vi "ParseOutput.vi"(8 "error in (no error)":errorcluster, 10 "JUnit report path":path, 11 "utf results in":T1[](array[typedef])) -> (0 "error out":errorcluster, 2 "Passed?":bool, 3 "Output":string)   [LabVIEW 2014, in "RunUnitTests.lvclass"]
uses:
  RunUnitTests.lvclass
  <vilib>/utf/common/utf_test_result_testfile.ctl
  <vilib>/utf/common/utf_test_result_testcase.ctl
  <vilib>/utf/common/utf_test_result.ctl
  <vilib>/utf/common/utf_test_result_troll_new.ctl
  <vilib>/utf/common/utf_vector_result.ctl
  <vilib>/utf/common/utf_test_result_failure.ctl
  <vilib>/utf/common/utf_test_comparison_operators.ctl
  <vilib>/utf/common/utf_vi_tag.ctl
  <vilib>/utf/common/utf_test_result_input_data.ctl
  <vilib>/utf/common/utf_code_coverage.ctl
  <vilib>/utf/common/utf_error_data.ctl
  <vilib>/utf/common/utf_error_type.ctl
  <vilib>/utf/common/utf_subvi_info.ctl
  <vilib>/utf/NI_UnitTestFramework.lvlib
panel:
  in  "JUnit report path infromation":string="Please find the JUnit report path at \"%s\"."
  in  "No of test path not processed":string="%d tests path not processed.\\n"
  in  "No of test path skipped":string="%d tests path skipped.\\n"
  in  "No of test path errored":string="%d tests path errored.\\n"
  in  "No of test path failed":string="%d tests path failed.\\n"
  in  "Number of test path passed":string="%d tests path passed.\\n"
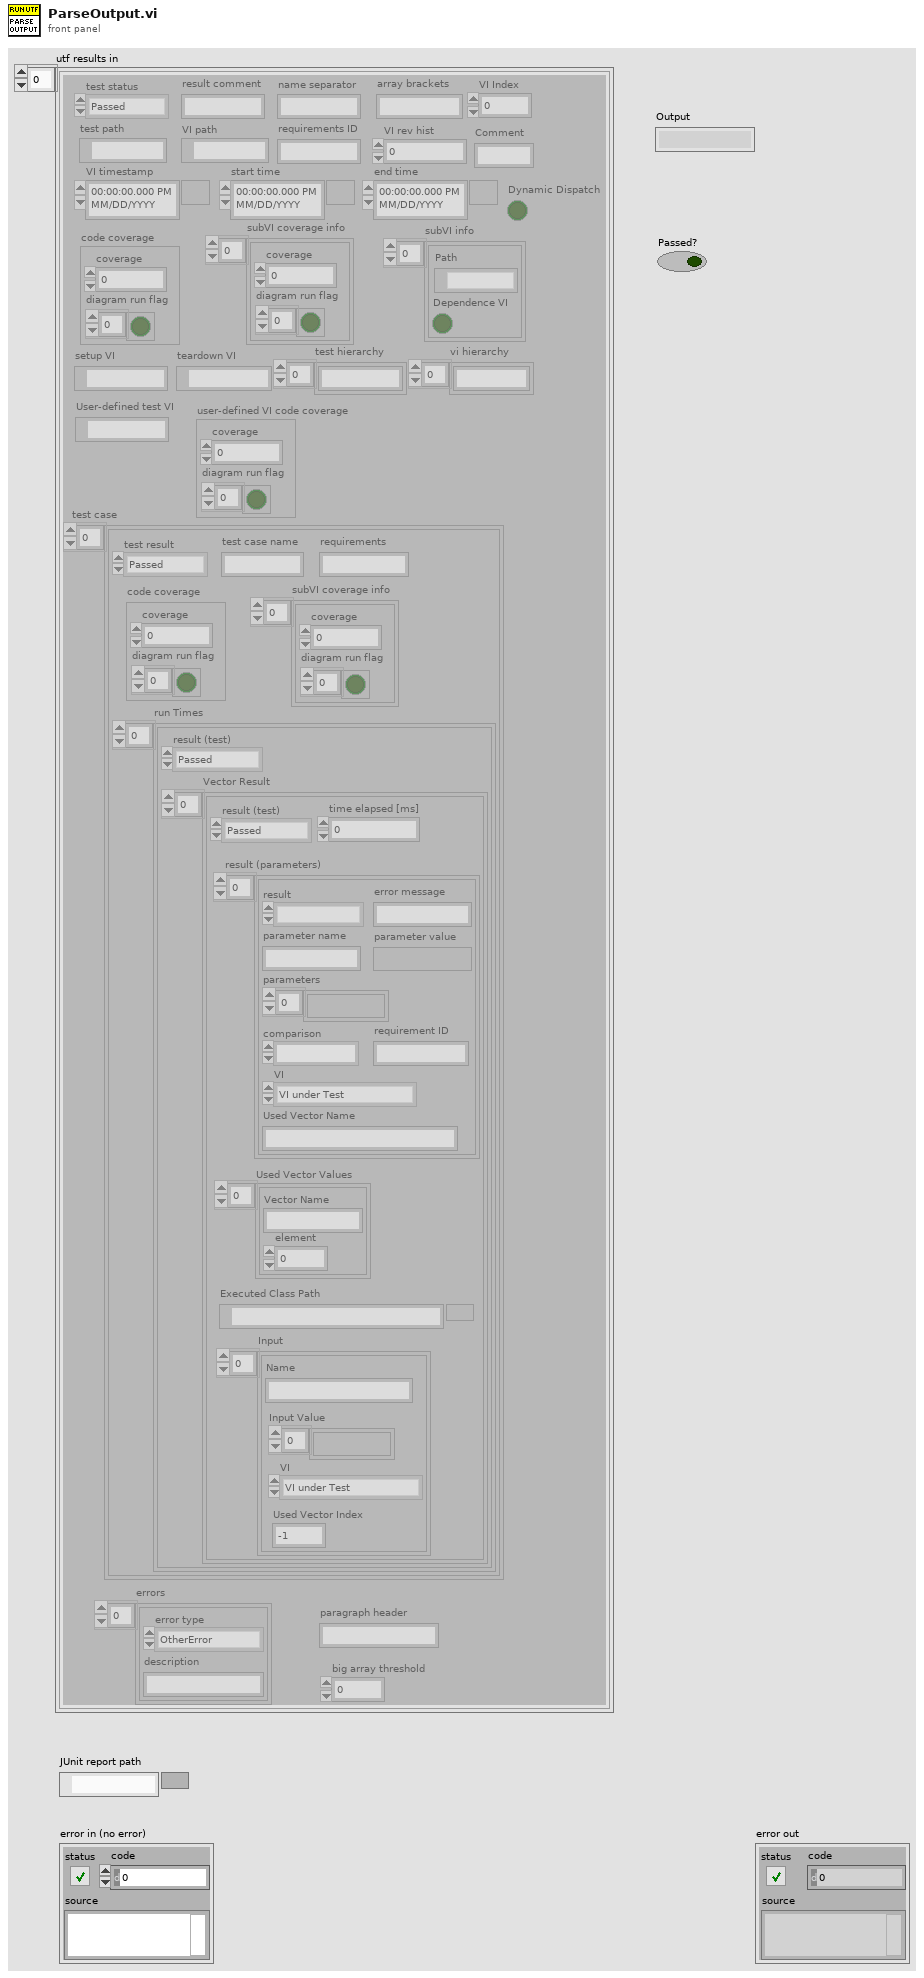
[diagram p1: front panel]
types:
  T1 = typedef "NI_UnitTestFramework.lvlib/utf_test_result_testfile.ctl" = cluster{"test case":T2[], "test status":T3, "test path":path, "setup VI":path, "teardown VI":path, "code coverage":T10, "start time":timestamp, "end time":timestamp, "test hierarchy":string[], "VI path":path, "VI timestamp":timestamp, "VI rev hist":i32, "requirements ID":string, "array brackets":string, "name separator":string, "errors":T11[], "paragraph header":string, "result comment":string, "vi hierarchy":string[], "subVI coverage info":T10[], "subVI info":T13[], "big array threshold":u32, "VI Index":i32, "Comment":string, "Dynamic Dispatch":bool, "User-defined test VI":path, "user-defined VI code coverage":T10}
  T2 = typedef "NI_UnitTestFramework.lvlib/utf_test_result_testcase.ctl" = cluster{"test result":T3, "run Times":T4[], "test case name":string, "requirements":string, "code coverage":T10, "subVI coverage info":T10[]}
  T3 = typedef "NI_UnitTestFramework.lvlib/utf_test_result.ctl" = enum16{"Passed", "Failed", "Error", "Skipped", "Not Processed"}
  T4 = typedef "NI_UnitTestFramework.lvlib/utf_test_result_troll_new.ctl" = cluster{"result (test)":T3, "Vector Result":T5[]}
  T5 = typedef "NI_UnitTestFramework.lvlib/utf_vector_result.ctl" = cluster{"time elapsed [ms]":u32, "result (test)":T3, "result (parameters)":T6[], "Used Vector Values":cluster{"Vector Name":string, "element":i32}[], "Executed Class Path":path, "Input":T9[]}
  T6 = typedef "NI_UnitTestFramework.lvlib/utf_test_result_failure.ctl" = cluster{"result":T3, "error message":string, "parameter name":string, "parameter value":variant, "parameters":variant[], "comparison":T7, "requirement ID":string, "VI":T8, "Used Vector Name":string}
  T7 = typedef "NI_UnitTestFramework.lvlib/utf_test_comparison_operators.ctl" = enum16{"=", "!=", ">", ">=", "<", "<=", "range", "symmetric tolerance", "asymmetric tolerance", "string contains", "string not contain", "array size", "string length", "array range", "by element", "array range (limit array)", "user-defined", "array contains", "array not contain", "vector length", "= (elm)", "!= (elm)", "= (case insensitive)", "!= (case insensitive)"}
  T8 = typedef "NI_UnitTestFramework.lvlib/utf_vi_tag.ctl" = enum16{"Setup VI", "VI under Test", "Teardown VI"}
  T9 = typedef "NI_UnitTestFramework.lvlib/utf_test_result_input_data.ctl" = cluster{"Name":string, "Input Value":variant[], "VI":T8, "Used Vector Index":i32}
  T10 = typedef "NI_UnitTestFramework.lvlib/utf_code_coverage.ctl" = cluster{"coverage":dbl, "diagram run flag":bool[]}
  T11 = typedef "NI_UnitTestFramework.lvlib/utf_error_data.ctl" = cluster{"error type":T12, "description":string}
  T12 = typedef "NI_UnitTestFramework.lvlib/utf_error_type.ctl" = enum16{"TestFileError", "VIError", "SetupVIError", "TearDownVIError", "OtherError"}
  T13 = typedef "NI_UnitTestFramework.lvlib/utf_subvi_info.ctl" = cluster{"Path":path, "Dependence VI":bool}
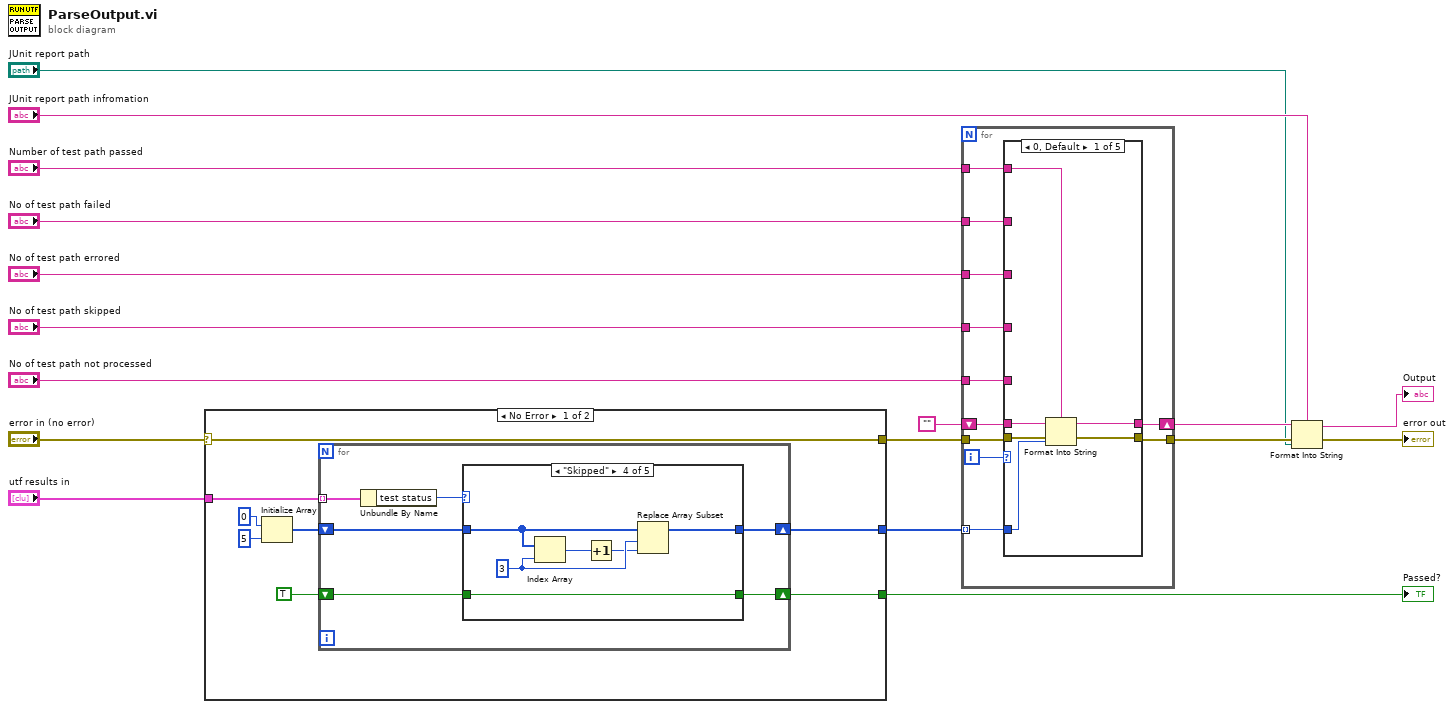
[diagram p0: block diagram]
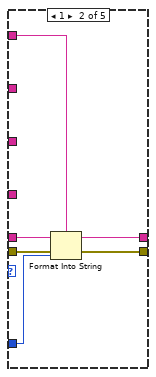
[diagram p2: hidden frame]
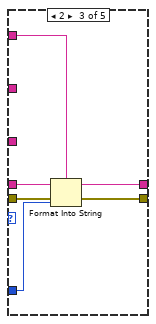
[diagram p3: hidden frame]
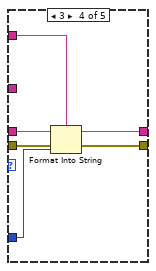
[diagram p4: hidden frame]
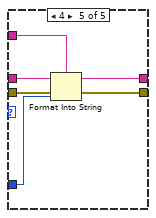
[diagram p5: hidden frame]
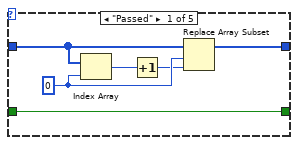
[diagram p6: hidden frame]
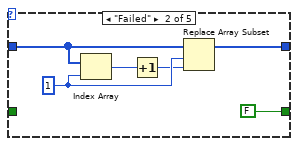
[diagram p7: hidden frame]
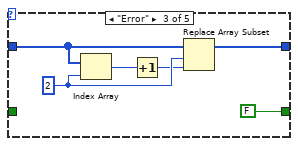
[diagram p8: hidden frame]
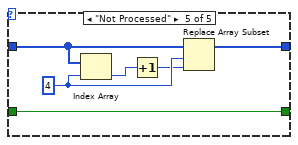
[diagram p9: hidden frame]
diagram:
  n1 = case shown="No Error" "error in (no error)" {
    selector: "error in (no error)" -> [w21 w62]
    tunnel: "utf results in" -> [w24 _]
    tunnel: [w22 _] -> w13
    tunnel: [w18 _] -> w15
    tunnel: [w21 w62] -> w14
    frame No Error {
      n2 = Initialize Array(0, 5 ("dimension size")) -> (w23:i32[])
      n3 = for {
        tunnel: w24 -> [w31] mode=indexing
        shift-right: [w29] -> w22
        shift-left: TRUE -> [w28]
        shift-right: [w26] -> w18
        shift-left: w23 -> [w27]
        n4 = Unbundle By Name(w31) -> ("test status"=w30:T3)
        n5 = case shown="\"Skipped\"" w30 {
          tunnel: [w36 FALSE FALSE w50 w56] -> w29
          tunnel: w28 -> [w36 _ _ w50 w56]
          tunnel: w27 -> [w35 w40 w46 w52 w58]
          tunnel: [w32 w38 w45 w51 w57] -> w26
          frame "Passed" {
            w34 = 0 ("index")
            n6 = Index Array(array=w35, index=w34) -> (element=w37:i32)
            n7 = Increment(x=w37) -> (x+1=w33:i32)
            n8 = Replace Array Subset(array=w35, new element=w33, index=w34) -> (w32:i32[])
          }
          frame "Failed" {
            w42 = 1 ("index")
            n9 = Index Array(array=w40, index=w42) -> (element=w43:i32)
            n10 = Increment(x=w43) -> (x+1=w41:i32)
            n11 = Replace Array Subset(array=w40, new element=w41, index=w42) -> (w38:i32[])
          }
          frame "Error" {
            w48 = 2 ("index")
            n12 = Index Array(array=w46, index=w48) -> (element=w49:i32)
            n13 = Increment(x=w49) -> (x+1=w47:i32)
            n14 = Replace Array Subset(array=w46, new element=w47, index=w48) -> (w45:i32[])
          }
          frame "Skipped" {
            w54 = 3 ("index")
            n15 = Index Array(array=w52, index=w54) -> (element=w55:i32)
            n16 = Increment(x=w55) -> (x+1=w53:i32)
            n17 = Replace Array Subset(array=w52, new element=w53, index=w54) -> (w51:i32[])
          }
          frame "Not Processed" {
            w60 = 4 ("index")
            n18 = Index Array(array=w58, index=w60) -> (element=w61:i32)
            n19 = Increment(x=w61) -> (x+1=w59:i32)
            n20 = Replace Array Subset(array=w58, new element=w59, index=w60) -> (w57:i32[])
          }
        }
      }
    }
    frame Error {
    }
  }
  "Passed?" <- w13
  n21 = for {
    tunnel: w15 -> [w63] mode=indexing
    shift-right: [w73] -> w5
    shift-left: "" -> [w72]
    tunnel: w14 -> [w71]
    tunnel: [w70] -> w4
    tunnel: "Number of test path passed" -> [w69]
    tunnel: "No of test path failed" -> [w68]
    tunnel: "No of test path errored" -> [w67]
    tunnel: "No of test path skipped" -> [w66]
    tunnel: "No of test path not processed" -> [w65]
    i -> [w64]
    n22 = case shown="0, Default" w64 {
      tunnel: [w79 w83 w91 w95 w101] -> w73
      tunnel: w72 -> [w78 w84 w88 w96 w102]
      tunnel: w71 -> [w77 w85 w89 w97 w103]
      tunnel: [w76 w82 w90 w94 w100] -> w70
      tunnel: w69 -> [w75 _ _ _ _]
      tunnel: w68 -> [_ w81 _ _ _]
      tunnel: w67 -> [_ _ w87 _ _]
      tunnel: w66 -> [_ _ _ w93 _]
      tunnel: w65 -> [_ _ _ _ w99]
      tunnel: w63 -> [w74 w80 w86 w92 w98]
      frame 0, Default {
        n23 = Format Into String(format string=w75, initial string=w78, error in=w77, w74) -> (resulting string=w79:string, error out=w76:errorcluster)
      }
      frame 1 {
        n24 = Format Into String(format string=w81, initial string=w84, error in=w85, w80) -> (resulting string=w83:string, error out=w82:errorcluster)
      }
      frame 2 {
        n25 = Format Into String(format string=w87, initial string=w88, error in=w89, w86) -> (resulting string=w91:string, error out=w90:errorcluster)
      }
      frame 3 {
        n26 = Format Into String(format string=w93, initial string=w96, error in=w97, w92) -> (resulting string=w95:string, error out=w94:errorcluster)
      }
      frame 4 {
        n27 = Format Into String(format string=w99, initial string=w102, error in=w103, w98) -> (resulting string=w101:string, error out=w100:errorcluster)
      }
    }
  }
  n28 = Format Into String(format string="JUnit report path infromation", initial string=w5, error in=w4, "JUnit report path") -> (resulting string=→"Output":string, error out=→"error out":errorcluster)
